vi "Create from Session.vi"(8 "Error In":errorcluster, 11 "Session In":refnum<class "Session.lvclass">) -> (0 "Error Out":errorcluster, 2 "File Info":refnum<class "File Info.lvclass">, 3 "Session Out":refnum<class "Session.lvclass">)   [LabVIEW 2018, in "Toolkit.lvlib" / "File Info.lvclass"]
uses:
  File Info.lvclass
  Session/Session.lvclass
  Session/Session.lvclass/Session.ctl
  SSH/SSH.lvclass
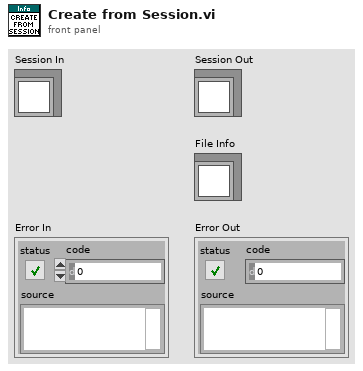
[diagram p1: front panel]
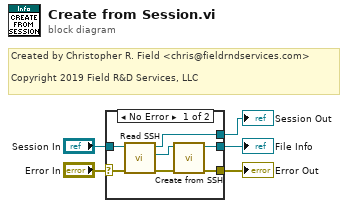
[diagram p0: block diagram]
diagram:
  # "Created by Christopher R. Field <chris@fieldrndservices.com>\n\nCopyright 2019 Field R&D Services, LLC"
  n1 = case shown="No Error" "Error In" {
    selector: "Error In" -> [w11 w14]
    tunnel: [w6 w14] -> w4
    tunnel: "Session In" -> [w12 w13]
    tunnel: [w9 w13] -> w2
    tunnel: [w8 _] -> w1
    frame No Error {
      n2 = call "Read SSH.vi"("Error In"=w11, "Session In"=w12) -> ("Erorr Out"=w7:errorcluster, "SSH"=w10:refnum<class "SSH.lvclass">, "Session Out"=w9:refnum<class "Session.lvclass">)  [unwired: 7 in]
      n3 = call "Create from SSH.vi"("Error In"=w7, "SSH"=w10) -> ("Error Out"=w6:errorcluster, "File Info"=w8:refnum<class "File Info.lvclass">)  [unwired: 8 in]
    }
    frame Error {
    }
  }
  "Error Out" <- w4
  "File Info" <- w1
  "Session Out" <- w2
